vi "test1.vi"() -> ()   [LabVIEW 2018]
panel:
  in  "camera mode":bool
  in  "gripper":i32(slide) scale=-125.0..125.0
  in  "grip":bool
  in  "base":i32(slide) scale=-125.0..125.0
  in  "speed 1":i32
  in  "step":dbl
  in  "z2":dbl
  in  "z1":dbl
  in  "x":dbl
  in  "stop":bool
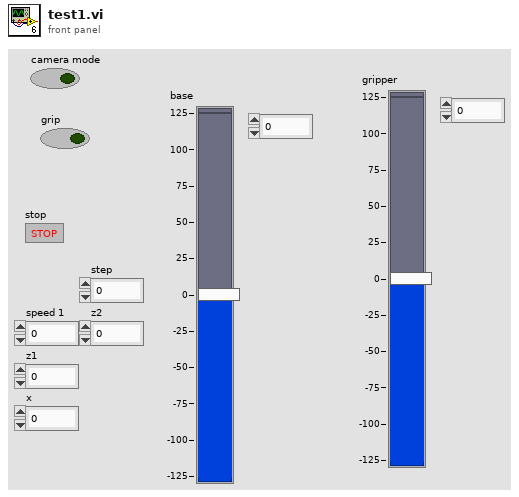
[diagram p1: front panel]
types:
  T1 = enum16{"shoulder", "elbow", "wrist", "base", "gripper"}
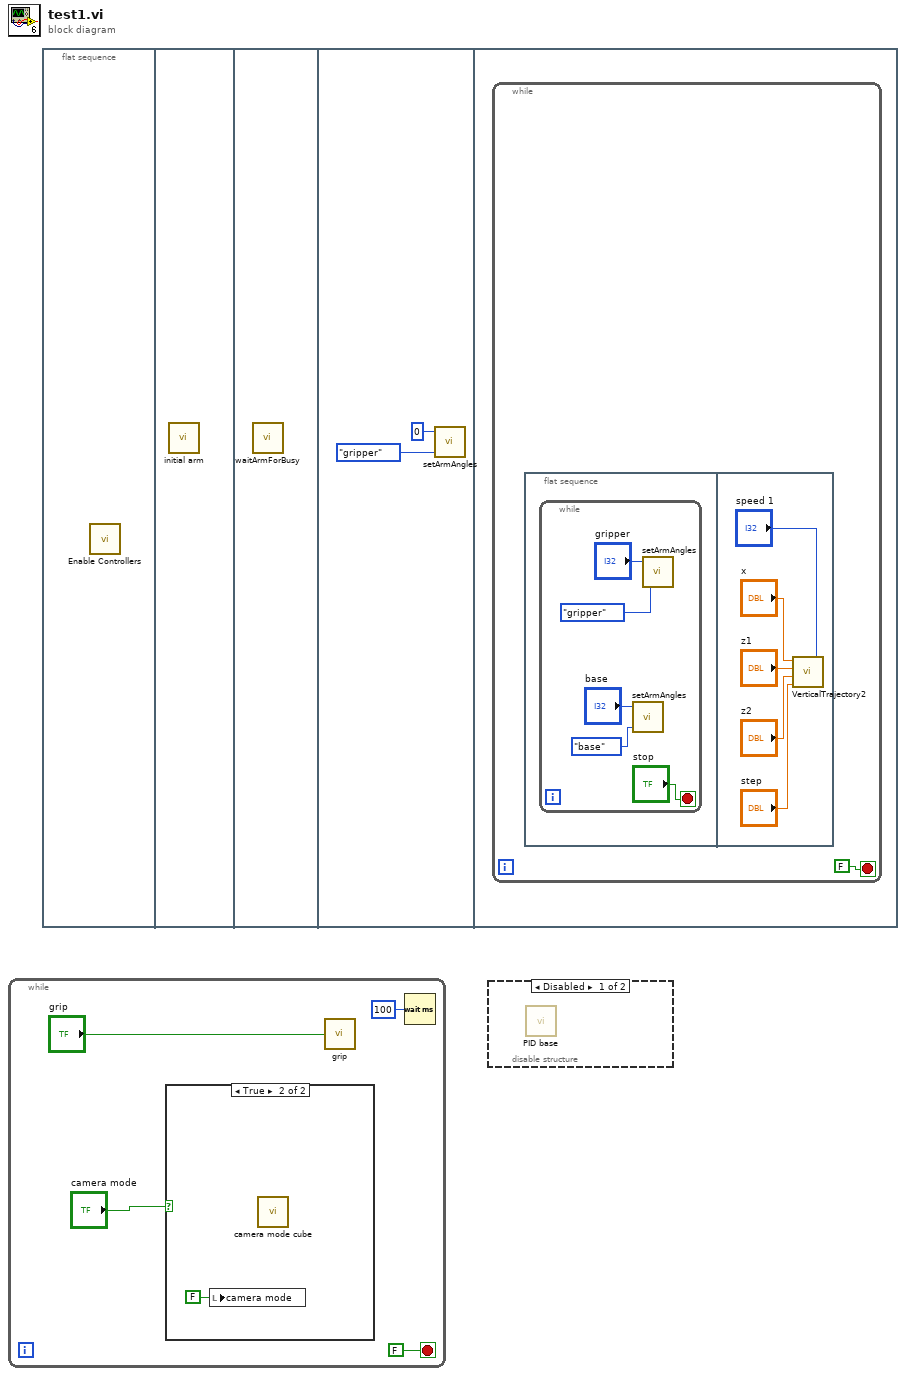
[diagram p0: block diagram]
diagram:
  n1 = while {
    stop <- FALSE stop-if-true
    n2 = case shown="True" "camera mode" {
      frame False {
      }
      frame True {
        n3 = local write "camera mode"(FALSE ("camera mode")) -> ()
        n4 = call "camera mode cube.vi"() -> ()  [unwired: 12 in]
      }
    }
    n5 = call "grip.vi"("grip"="grip") -> ()
    n6 = Wait (ms)(milliseconds to wait=u32 100) -> ()  [unwired: 1 out]
  }
  n7 = flat-sequence {
    frame #0 {
      n8 = call "Enable Controllers.vi"() -> ()  [unwired: 12 in]
    }
    frame #1 {
      n9 = call "initial arm.vi"() -> ()  [unwired: 12 in]
    }
    frame #2 {
      n10 = call "waitArmForBusy.vi"() -> ()  [unwired: 12 in]
    }
    frame #3 {
      n11 = call "setArmAngles.vi"("Enum"=T1."gripper", "angle"=0) -> ()  [unwired: 2 in]
    }
    frame #4 {
      n12 = while {
        stop <- FALSE stop-if-true
        n13 = flat-sequence {
          frame #0 {
            n14 = while {
              stop <- "stop" stop-if-true
              n15 = call "setArmAngles.vi"("Enum"=enum16{"shoulder", "elbow", "wrist", "base"}."base", "angle"="base") -> ()  [unwired: 2 in]
              n16 = call "setArmAngles.vi"("Enum"=T1."gripper", "angle"="gripper") -> ()  [unwired: 2 in]
            }
          }
          frame #1 {
            n17 = call "VerticalTrajectory2.vi"("speed 1"="speed 1", "step"="step", "z2"="z2", "z1"="z1", "x"="x") -> ()  [unwired: 3 in]
          }
        }
      }
    }
  }
  n18 = disable-structure shown="Disabled" {
    frame Disabled {
      n19 = call "PID base.vi"() -> ()  [unwired: 12 in]
    }
    frame Enabled {
    }
  }
